vi "Create Listener.vi"(8 "error in (no error)":errorcluster, 11 "TCP Server in":refnum<class "TCP Server.lvclass">) -> (0 "error out":errorcluster, 3 "TCP Server out":refnum<class "TCP Server.lvclass">)   [LabVIEW 2024, in "Stream-TCP.lvlib" / "TCP Server.lvclass"]
uses:
  TCP Server.lvclass
  C:/dev/lv20CE/relink/lv-stream/stream/Endpoint/Endpoint.lvclass
  TCP Server.lvclass/TCP Server.ctl
  lv-stream/stream/Endpoint/Endpoint.lvclass
  lv-stream/stream/URI/URI.lvclass
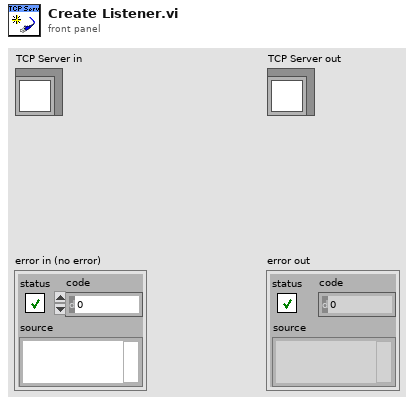
[diagram p1: front panel]
types:
  T1 = typedef "Stream-TCP.lvlib/TCP Server.lvclass/Ref Data.ctl" = cluster{"Listener":refnum<k5>, "Clients":refnum<class "TCP Client.lvclass">[], "Server Loop":bool}
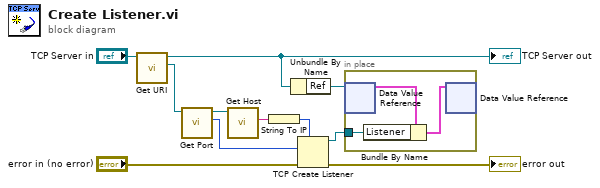
[diagram p0: block diagram]
diagram:
  n1 = call "Get URI.vi"("Endpoint in"="TCP Server in") -> ("URI"=w10:refnum<class "URI.lvclass">, "Endpoint out"=w2:refnum<class "TCP Server.lvclass">)  [unwired: 8 in, 1 out]
  "TCP Server out" <- w2
  n2 = call "Get Port.vi"("URI in"=w10) -> ("Port"=w6:u16, "URI out"=w9:refnum<class "URI.lvclass">)  [unwired: 8 in, 1 out]
  n3 = call "Get Host.vi"("URI in"=w9) -> ("Host"=w8:string)  [unwired: 8 in, 2 out]
  n4 = String To IP(1:w8) -> (0:w7:u32)
  n5 = Unbundle By Name(w2) -> ("Ref"=w4:refnum<data-value>)
  n6 = TCP Create Listener(7:w7, 8:"error in (no error)", 10:w6) -> (0:→"error out":errorcluster, 3:w3:refnum<k5>)  [unwired: 2 in, 1 out]
  n7 = in-place {
    in-place-border: w3 -> [w12]
    n8 = in-place-dvr #1(w4) -> (w14:T1)  [unwired: 1 out]
    n9 = Bundle By Name(cluster=w14, "Listener"=w12) -> (w13:T1)
    n10 = in-place-dvr #1(w13) -> ()  [unwired: 2 out]
  }
